vi "Read_relay.vi"() -> (1 "unsigned 8bit integer":u8, 2 "Boolean array":bool[](array[boolean]))   [LabVIEW 2019]
uses:
  D2XX_Functions/D2XX_Functions.lvlib
panel:
  out "error out":errorcluster
  in  "error in (no error)":errorcluster
  out "FT_Status":u32(ring) items=["FT_OK", "FT_INVALID_HANDLE", "FT_DEVICE_NOT_FOUND", "FT_DEVICE_NOT_OPENED", "FT_IO_ERROR", "FT_INSUFFICIENT_RESOURCES", "FT_INVALID_PARAMETER", "FT_INVALID_BAUD_RATE", "FT_DEVICE_NOT_OPENED_FOR_ERASE", "FT_DEVICE_NOT_OPENED_FOR_WRITE", "FT_FAILED_TO_WRITE_DEVICE", "FT_EEPROM_READ_FAILED", "FT_EEPROM_WRITE_FAILED", "FT_EEPROM_ERASE_FAILED", "FT_EEPROM_NOT_PRESENT", "FT_EEPROM_NOT_PROGRAMMED", "FT_INVALID_ARGS", "FT_NOT_SUPPORTED", "FT_OTHER_ERROR"]
  out "Port Index":string
  out "Device Description":string
  out "FT_Status 2":u32(ring) items=["FT_OK", "FT_INVALID_HANDLE", "FT_DEVICE_NOT_FOUND", "FT_DEVICE_NOT_OPENED", "FT_IO_ERROR", "FT_INSUFFICIENT_RESOURCES", "FT_INVALID_PARAMETER", "FT_INVALID_BAUD_RATE", "FT_DEVICE_NOT_OPENED_FOR_ERASE", "FT_DEVICE_NOT_OPENED_FOR_WRITE", "FT_FAILED_TO_WRITE_DEVICE", "FT_EEPROM_READ_FAILED", "FT_EEPROM_WRITE_FAILED", "FT_EEPROM_ERASE_FAILED", "FT_EEPROM_NOT_PRESENT", "FT_EEPROM_NOT_PROGRAMMED", "FT_INVALID_ARGS", "FT_NOT_SUPPORTED", "FT_OTHER_ERROR"]
  # "Discharge tip"
  # "0 ohm"
  # "100k ohm"
  # "10M ohm"
  # "1Gohm"
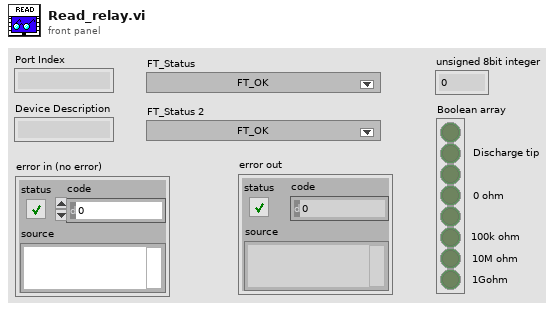
[diagram p1: front panel]
types:
  T1 = cluster{"Signature 1":u32, "Signature 2":u32, "Version":u32, "Vendor ID":u16, "Product ID":u16, "Manufacturer":string, "Manufacturer ID":string, "Description":string, "Serial Number":string, "Max Power (mA)":u16, "PnP":u16, "Self Powered":u16, "Remote Wake-Up":u16, "Rev4":u8, "Iso In":u8, "Iso Out":u8, "Pull Down Enable":u8, "Serial Number Enable":u8, "USB Version Enable":u8, "USB Version":u16, "Rev5":u8, "Iso In A":u8, "Iso In B":u8, "Iso Out A":u8, "Iso Out B":u8, "Pull Down Enable 5":u8, "Serial Number Enable 5":u8, "USB Version Enable 5":u8, "USB Version 5":u16, "A Is High Current":u8, "B Is High Current":u8, "A Is 245 FIFO":u8, "A Is CPU FIFO":u8, "A Is Fast Serial":u8, "A Is VCP":u8, "B Is 245 FIFO":u8, "B Is CPU FIFO":u8, "B Is Fast Serial":u8, "B Is VCP":u8, "Use Ext Osc":u8, "High Drive IOs":u8, "Endpoint Size":u8, "Pull Down Enable R":u8, "Serial Number Enable R":u8, "Invert TXD":u8, "Invert RXD":u8, "Invert RTS":u8, "Invert CTS":u8, "Invert DTR":u8, "Invert DSR":u8, "Invert DCD":u8, "Invert RI":u8, "CBus0":u8, "CBus1":u8, "CBus2":u8, "CBus3":u8, "CBus4":u8, "R Is VCP":u8, "Pull Down Enable 7":u8, "Serial Number Enable 7":u8, "AL Slow Slew":u8, "AL Schmitt Input":u8, "AL Drive Current":u8, "AH Slow Slew":u8, "AH Schmitt Input":u8, "AH Drive Current":u8, "BL Slow Slew":u8, "BL Schmitt Input":u8, "BL Drive Current":u8, "BH Slow Slew":u8, "BH Schmitt Input":u8, "BH Drive Current":u8, "A Is 245 FIFO 7":u8, "A Is CPU FIFO 7":u8, "A Is Fast Serial 7":u8, "A Is VCP 7":u8, "B Is 245 FIFO 7":u8, "B Is CPU FIFO 7":u8, "B Is Fast Serial 7":u8, "B Is VCP 7":u8, "PowerSaveEnable":u8, "Pull Down Enable 8":u8, "Serial Number Enable 8":u8, "A Slow Slew":u8, "A Schmitt Input":u8, "A Drive Current":u8, "B Slow Slew":u8, "B Schmitt Input":u8, "B Drive Current":u8, "C Slow Slew":u8, "C Schmitt Input":u8, "C Drive Current":u8, "D Slow Slew":u8, "D Schmitt Input":u8, "D Drive Current":u8, "A RI Is TXDEN":u8, "B RI Is TXDEN":u8, "C RI Is TXDEN":u8, "D RI Is TXDEN":u8, "A Is VCP 8":u8, "B Is VCP 8":u8, "C Is VCP 8":u8, "D Is VCP 8":u8}
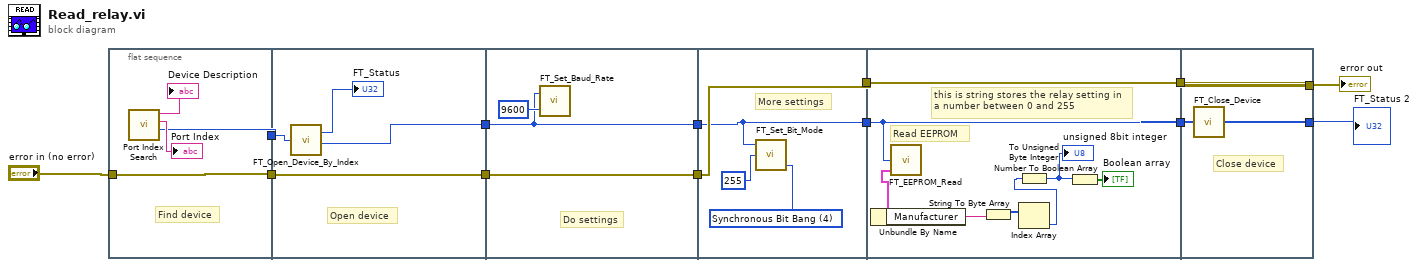
[diagram p0: block diagram]
diagram:
  n1 = flat-sequence {
    tunnel: [w14] -> w13
    tunnel: "error in (no error)" -> [w15]
    tunnel: [w15] -> w12
    tunnel: w13 -> [w20]
    tunnel: [w18] -> w11
    tunnel: [w19] -> w10
    tunnel: w12 -> [w19]
    tunnel: [w22] -> w9
    tunnel: w11 -> [w22]
    tunnel: [w23] -> w8
    tunnel: w10 -> [w23]
    tunnel: w9 -> [w25]
    tunnel: w8 -> [w26]
    tunnel: [w26] -> w4
    tunnel: [w25] -> w3
    tunnel: [w31] -> w2
    tunnel: w4 -> [w36]
    tunnel: [w36] -> w1
    tunnel: w3 -> [w31]
    tunnel: w2 -> [w38]
    tunnel: [w39] -> w7
    tunnel: [w37] -> w5
    tunnel: w1 -> [w37]
    frame #0 {
      # "Find device"
      n2 = call "Port Index Search.vi"() -> ("Decimal Port Index"=w14:i32, "Port Index"=→"Port Index":string, "Device Description"=→"Device Description":string)  [unwired: 8 in, 1 out]
    }
    frame #1 {
      # "Open device"
      n3 = call "FT_Open_Device_By_Index.vi"("Device Index"=w20) -> ("FT_Status"=→"FT_Status":u32, "Handle"=w18:u32)
    }
    frame #2 {
      # "Do settings"
      n4 = call "FT_Set_Baud_Rate.vi"("Baud Rate"=u32 9600, "Handle"=w22) -> ()  [unwired: 1 out]
    }
    frame #3 {
      w28 = u8 4 items=["Reset Bit Mode"=0, "Asynchronous Bit Bang"=1, "MPSSE"=2, "Synchronous Bit Bang"=4, "MCU Host Bus Emulation"=8, "Fast Opto-Isolated Serial"=16, "CBUS Bit Bang"=32, "Single Channel 245 Synchronous FIFO"=64] ("Bit Mode")
      # "More settings"
      n5 = call "FT_Set_Bit_Mode.vi"("Bit Mode"=w28, "Bit Mode Mask"=u8 255, "Handle"=w25) -> ()  [unwired: 1 out]
    }
    frame #4 {
      # "Read EEPROM"
      # "this is string stores the relay setting in\na number between 0 and 255"
      n6 = call "FT_EEPROM_Read.vi"("Handle"=w31) -> ("output cluster"=w35:T1)  [unwired: 2 out]
      n7 = Unbundle By Name(w35) -> ("Manufacturer"=w34:string)
      n8 = String To Byte Array(string=w34) -> (unsigned byte array=w33:u8[])
      n9 = Index Array(array=w33) -> (element=w32:u8)  [unwired: 1 in]
      n10 = To Unsigned Byte Integer(number=w32) -> (unsigned 8bit integer=w30:u8)
      "unsigned 8bit integer" <- w30
      n11 = Number To Boolean Array(number=w30) -> (Boolean array=→"Boolean array":bool[])
    }
    frame #5 {
      # "Close device"
      n12 = call "FT_Close_Device.vi"("Handle"=w38) -> ("FT_Status"=w39:u32)
    }
  }
  "FT_Status 2" <- w7
  "error out" <- w5
